vi "Set_SglVar_Value.vi"(8 "error in (no error)":errorcluster, 9 "varValue":dbl format="%#_13g", 11 "muExpr in":refnum<class "mupExpr.lvclass">) -> (0 "error out":errorcluster, 3 "muExpr out":refnum<class "mupExpr.lvclass">)   [LabVIEW 2015, in "mupExpr.lvclass"]
doc: "Set the value of the expression's single variable.\n\nIf the expression contains no variables, the input value is ignored."
uses:
  mupExpr.lvclass
  mupExpr.lvclass/mupExpr.ctl
  mupLib/mupLib.lvlib
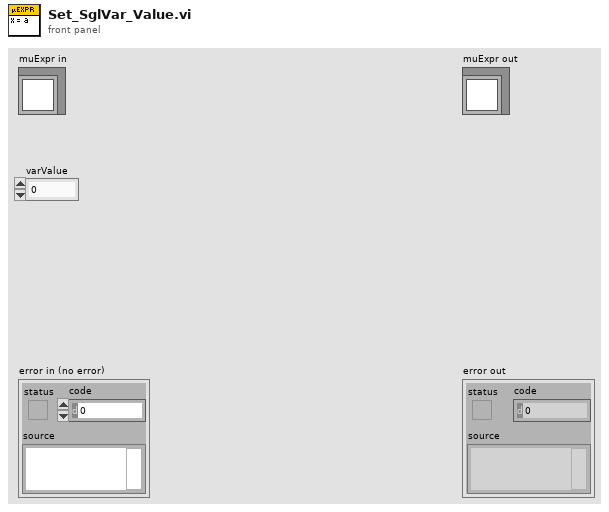
[diagram p1: front panel]
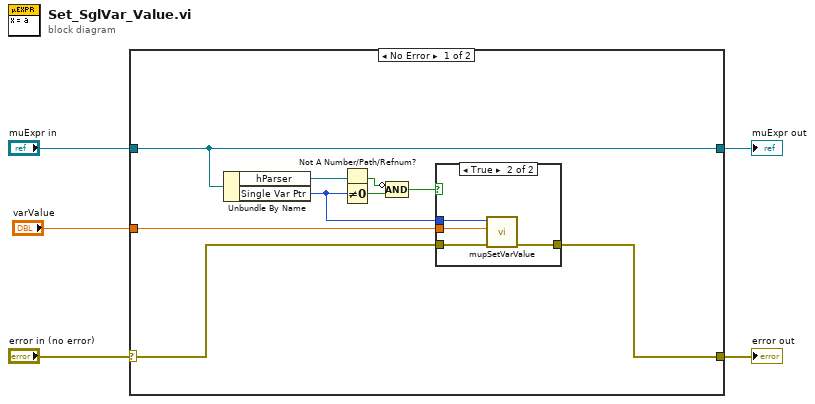
[diagram p0: block diagram]
diagram:
  n1 = case shown="No Error" "error in (no error)" {
    selector: "error in (no error)" -> [w11 w20]
    tunnel: "varValue" -> [w14 _]
    tunnel: "muExpr in" -> [w12 w21]
    tunnel: [w10 w20] -> w3
    tunnel: [w12 w21] -> w2
    frame No Error {
      n2 = Unbundle By Name(w12) -> ("hParser"=w7:refnum<data-value>, "Single Var Ptr"=w13:u64)
      n3 = Not A Number/Path/Refnum?(number/path/refnum=w7) -> (NaN/Path/Refnum?=w6:bool)
      n4 = Not Equal To 0?(x=w13) -> (x != 0?=w9:bool)
      n5 = Compound Arithmetic op=AND(invert w6, w9) -> (w8:bool)
      n6 = case shown="True" w8 {
        tunnel: w13 -> [_ w19]
        tunnel: w14 -> [_ w18]
        tunnel: w11 -> [w15 w17]
        tunnel: [w15 w16] -> w10
        frame False {
        }
        frame True {
          n7 = call "mupSetVarValue.vi"("error in (no error)"=w17, "varValue"=w18, "varAddr in"=w19) -> ("error out"=w16:errorcluster)  [unwired: 7 in, 1 out]
        }
      }
    }
    frame Error {
    }
  }
  "error out" <- w3
  "muExpr out" <- w2
